vi "NF87XX.absolute move.vi"(0 "i ref in":refnum<vi>, 1 "System":string="N/A", 2 "forward?":bool, 3 "velocity (1 .. 2000)":dbl=1.0 min=1.0 max=2000.0, 5 "error in (no error)":errorcluster) -> (14 "i ref out":refnum<vi>, 19 "error out":errorcluster)   [LabVIEW 2014, in "NF87XX.lvlib"]
doc: "This VI sets acceleration, velocity and goal position and starts the absolute move. Only possible for 1-channel closed loop driver systems.\n\nauthor: Stefan Götte\ndata: 09-JAN-2007\n\nLicense Agreement for this software:\n\nCopyright (C)\nGesellschaft für Schwerionenforschung, GSI\nPlanckstr. 1\n64291 Darmstadt\nGermany\n\nContact: D.Beck@gsi.de \n\nThis program is free software; you can redistribute it and/or modify it under the terms of the GNU General Public License as published by the Free Software Foundation; either version 2 of the license, or (at your option) any later version.\n\nThis program is distributed in the hope that it will be useful, but WITHOUT ANY WARRANTY; without even the implied warranty of MERCHANTABILITY or FITNESS FOR A PARTICULAR PURPOSE. See the GNU General License for more details (http://www.gnu.org).\n\nGesellschaft für Schwerionenforschung, GSI\nPlanckstr. 1, 64291 Darmstadt, Germany\nFor all questions and ideas contact: M.Richter@gsi.de, H.Brand@gsi.de or D.Beck@gsi.de.\nLast update: 17-JUN-2004"
uses:
  NF87XX.lvlib
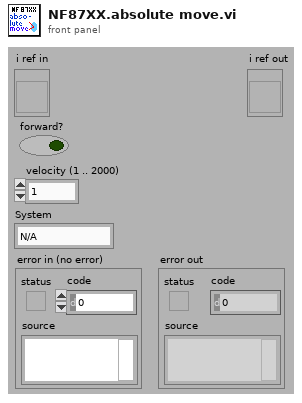
[diagram p1: front panel]
types:
  T1 = typedef "NF87XX.lvlib/NF87XX.driver Type.ctl" = enum16{"not defined", "3-ch open loop drv", "1-ch closed loop drv"}
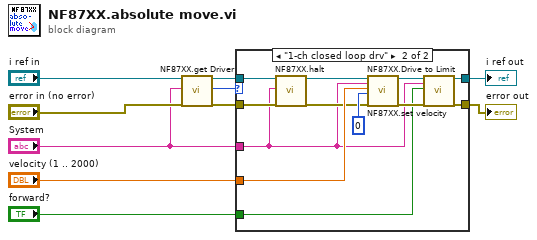
[diagram p0: block diagram]
diagram:
  n1 = call "NF87XX.get Driver.vi"("i ref in"="i ref in", "System"="System", "error in (no error)"="error in (no error)") -> ("i ref out"=w6:refnum<vi>, "Driver Type"=w1:T1, "error out"=w4:errorcluster)  [unwired: 12 in, 2 out]
  n2 = case shown="\"1-ch closed loop drv\"" w1 {
    tunnel: "forward?" -> [_ w13]
    tunnel: "velocity (1 .. 2000)" -> [_ w22]
    tunnel: [w12 w21] -> w8
    tunnel: [w11 w20] -> w7
    tunnel: w6 -> [w12 w16]
    tunnel: w4 -> [w11 w18]
    tunnel: "System" -> [_ w14]
    frame "not defined", Default {
    }
    frame "1-ch closed loop drv" {
      n3 = call "NF87XX.halt.vi"("i ref in"=w16, "System"=w14, "error in (no error)"=w18) -> ("i ref out"=w15:refnum<vi>, "error out"=w17:errorcluster)  [unwired: 15 in]
      n4 = call "NF87XX.set velocity.vi"("i ref in"=w15, "System"=w14, "velocity (1 .. 2000)"=w22, "Motor (0,1,2)"=0 ("Motor (0, 1 or 2)"), "error in (no error)"=w17) -> ("i ref out"=w23:refnum<vi>, "error out"=w24:errorcluster)  [unwired: 13 in]
      n5 = call "NF87XX.Drive to Limit.vi"("i ref in"=w23, "System"=w14, "Forward?"=w13, "error in (no error)"=w24) -> ("i ref out"=w21:refnum<vi>, "error out"=w20:errorcluster)  [unwired: 14 in]
    }
  }
  "error out" <- w7
  "i ref out" <- w8
